vi "Group_FromXML.vi"(8 "error in (no error)":errorcluster, 11 "XML String":string) -> (0 "error out":errorcluster, 3 "Group out":refnum<class "Group.lvclass">)   [LabVIEW 2023, in "Group.lvclass"]
doc: "Create the group definition based on a given XML string."
uses:
  Group.lvclass
  GroupAsCluster.ctl
  Channel/ChannelAsCluster.ctl
  <vilib>/NI VeriStand/Custom Device API/Data Reference.ctl
  Meta Data.ctl
  <vilib>/NI VeriStand/Custom Device API/Custom Device API.lvlib
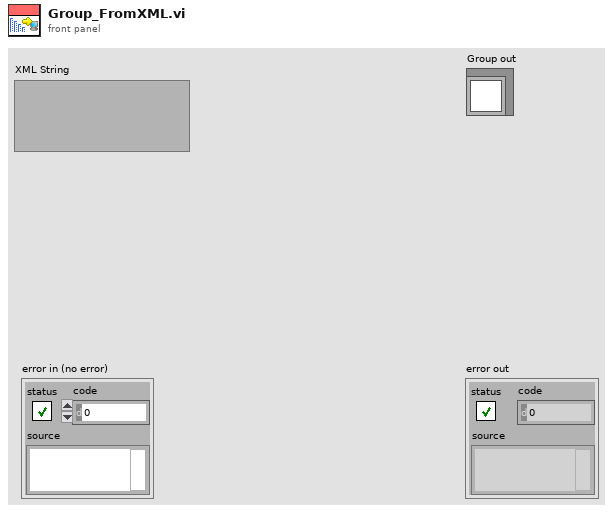
[diagram p1: front panel]
types:
  T1 = typedef "GroupAsCluster.ctl" = cluster{"Name":string, "Channels":T2[], "Meta Data":T4[]}
  T2 = typedef "ChannelAsCluster.ctl" = cluster{"Name":string, "Data Reference":T3, "Wfm?":bool, "Decimation":i32, "Current Value":dbl, "Meta Data":T4[], "WfmPath":string}
  T3 = typedef "Custom Device API.lvlib/Data Reference.ctl" = i32
  T4 = typedef "Meta Data.ctl" = cluster{"Key":string, "Value":string}
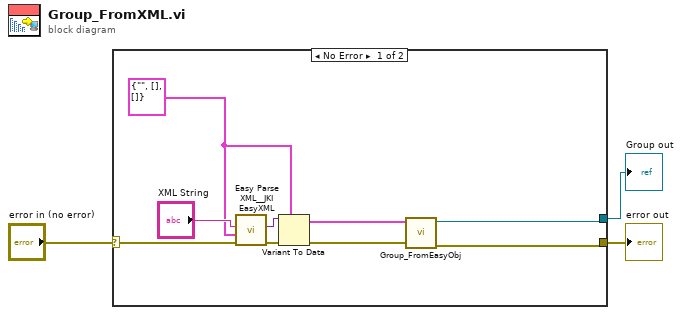
[diagram p0: block diagram]
diagram:
  n1 = case shown="No Error" "error in (no error)" {
    selector: "error in (no error)" -> [w9 w13]
    tunnel: [w4 w13] -> w2
    tunnel: [w5 _] -> w1
    frame No Error {
      w8 = T1 {"Name"="", "Channels"=[], "Meta Data"=[]} ("output cluster")
      n2 = call <vilib>:"Easy Parse XML__JKI EasyXML.vi"("error in (no error)"=w9, "LabVIEW Data (Type)"=w8, "XML String"="XML String") -> ("error out"=w10:errorcluster, "LabVIEW Data"=w11:variant)  [unwired: 7 in]
      n3 = Variant To Data(error in=w10, type=w8, Variant=w11) -> (data=w7:T1, error out=w6:errorcluster)
      n4 = call "Group_FromEasyObj.vi"("error in (no error)"=w6, "input cluster"=w7) -> ("error out"=w4:errorcluster, "Group out"=w5:refnum<class "Group.lvclass">)  [unwired: 8 in]
    }
    frame Error {
    }
  }
  "error out" <- w2
  "Group out" <- w1
